vi "ABB Norma 5000 Configure Input.vi"(5 "Current Shunt Factor":dbl=1.0 min=0.0 step=0.01 format="%.2f", 6 "Phase":i32=1, 7 "Current Shunt":i32(ring) items=["Internal", "External"], 8 "error in (no error)":errorcluster, 9 "Channel":i32(ring) items=["Current", "Voltage"], 10 "Coupling":i32(ring) items=["DC", "AC"], 11 "VISA session":refnum<visa-resource-name>) -> (0 "error out":errorcluster, 3 "dup VISA session":refnum<visa-resource-name>)   [LabVIEW 2017]
doc: "This VI configures the specified input of the instrument."
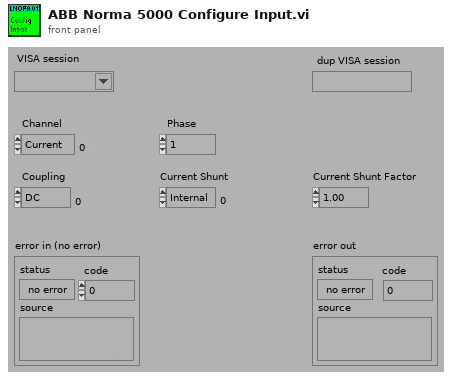
[diagram p1: front panel]
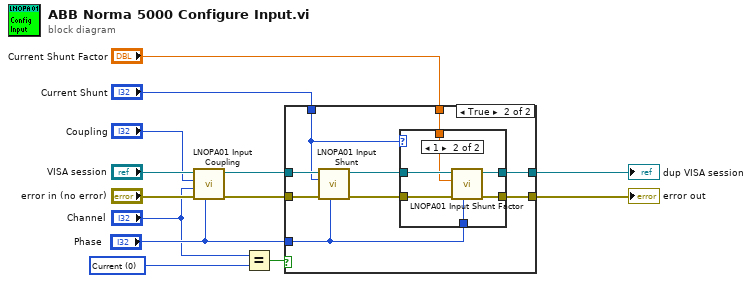
[diagram p0: block diagram]
diagram:
  w4 = 0 items=["Current", "Voltage"] ("Channel")
  n1 = call "LNOPA01 Input Coupling.vi"("Phase"="Phase", "error in (no error)"="error in (no error)", "Channel"="Channel", "Coupling"="Coupling", "VISA session"="VISA session") -> ("error out"=w10:errorcluster, "dup VISA session"=w11:refnum<visa-resource-name>)  [unwired: 4 in, 1 out]
  n2 = Equal?(x="Channel", y=w4) -> (x = y?=w3:bool)
  n3 = case shown="True" w3 {
    tunnel: w11 -> [w15 w24]
    tunnel: w10 -> [w14 w23]
    tunnel: [w15 w20] -> w2
    tunnel: [w14 w19] -> w1
    tunnel: "Phase" -> [_ w18]
    tunnel: "Current Shunt Factor" -> [_ w17]
    tunnel: "Current Shunt" -> [_ w16]
    frame False {
    }
    frame True {
      n4 = call "LNOPA01 Input Shunt.vi"("Phase"=w18, "error in (no error)"=w23, "Shunt"=w16, "VISA session"=w24) -> ("error out"=w21:errorcluster, "dup VISA session"=w22:refnum<visa-resource-name>)  [unwired: 5 in, 1 out]
      n5 = case shown="1" w16 {
        tunnel: w22 -> [w26 w32]
        tunnel: w21 -> [w25 w31]
        tunnel: [w26 w30] -> w20
        tunnel: [w25 w29] -> w19
        tunnel: w18 -> [_ w27]
        tunnel: w17 -> [_ w28]
        frame 0, Default {
        }
        frame 1 {
          n6 = call "LNOPA01 Input Shunt Factor.vi"("Phase"=w27, "error in (no error)"=w31, "Shunt Factor"=w28, "VISA session"=w32) -> ("error out"=w29:errorcluster, "dup VISA session"=w30:refnum<visa-resource-name>)  [unwired: 5 in, 1 out]
        }
      }
    }
  }
  "error out" <- w1
  "dup VISA session" <- w2
